vi "Base Json Pretty Formatter.vi"(8 "error in":errorcluster, 10 "ATS Framework Fields in":T1, 11 "json in":string) -> (0 "error out":errorcluster, 3 "json out":string)   [LabVIEW 2022 SP3]
uses:
  Arcadia/Common/Framework/ATS Framework Fields.ctl
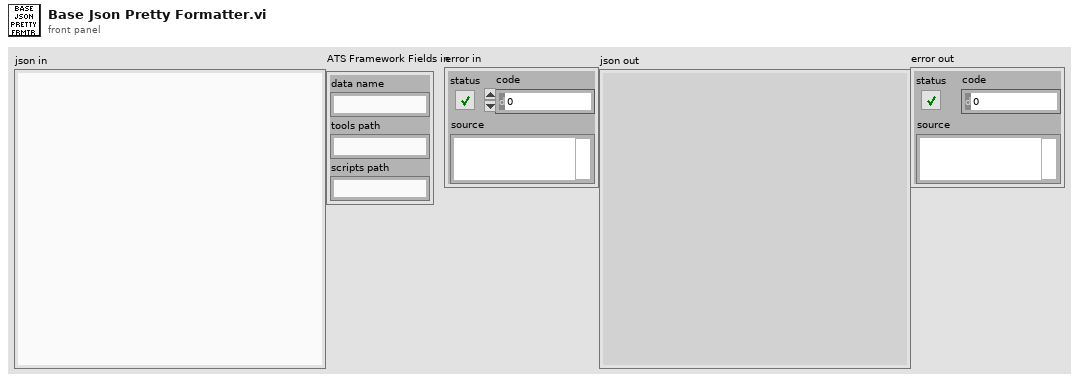
[diagram p1: front panel]
types:
  T1 = typedef "ATS Framework Fields.ctl" = cluster{"data name":string, "tools path":string, "scripts path":string}
  T2 = typedef "Run Tool Output.ctl" = cluster{"cmdline":string, "stdout":string, "stderr":string}
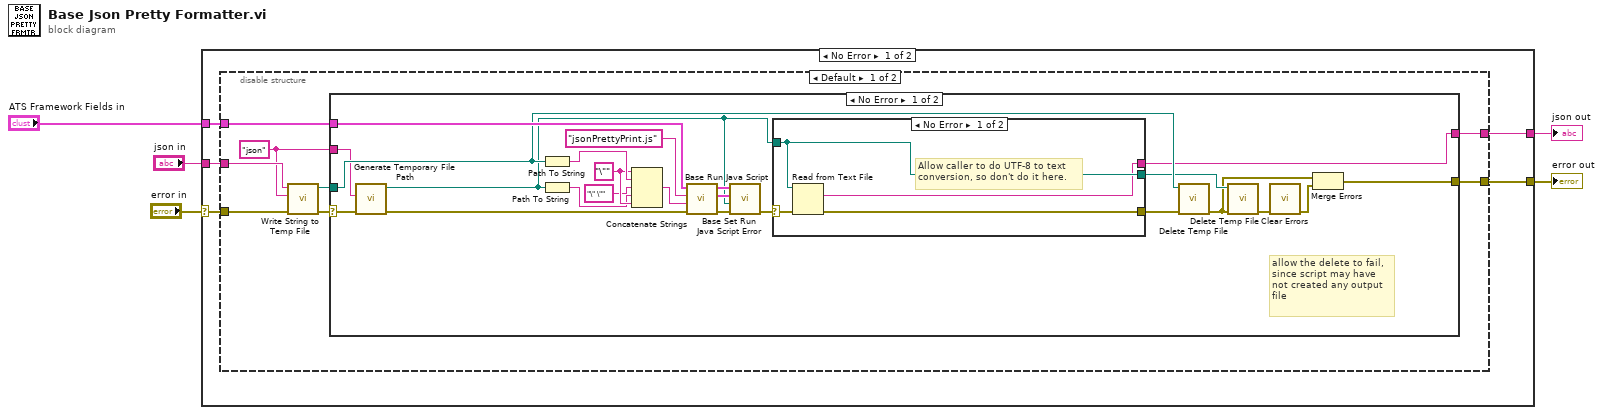
[diagram p0: block diagram]
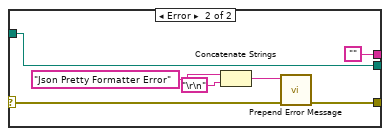
[diagram p2: hidden frame]
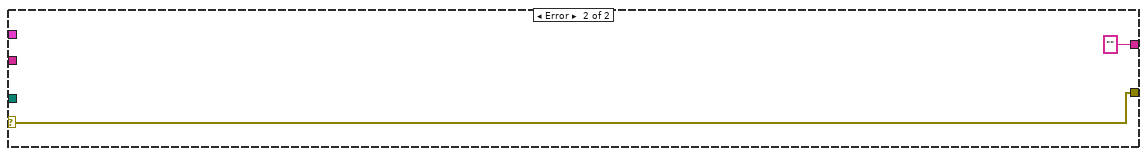
[diagram p3: hidden frame]
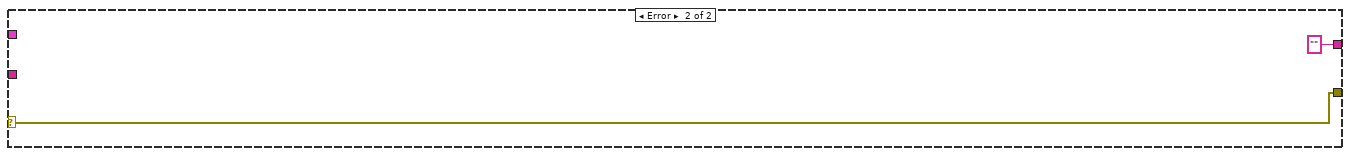
[diagram p5: hidden frame]
diagram:
  n1 = case shown="No Error" "error in" {
    selector: "error in" -> [w7 w58]
    tunnel: [w6 w58] -> w5
    tunnel: "ATS Framework Fields in" -> [w10 _]
    tunnel: [w9 "" ("std out")] -> w2
    tunnel: "json in" -> [w8 _]
    frame No Error {
      n2 = disable-structure shown="Default" {
        disable-tunnel: w10 -> [w18 _]
        disable-tunnel: [w17 w55] -> w9
        disable-tunnel: w8 -> [w16 w55]
        disable-tunnel: w7 -> [w15 w56]
        disable-tunnel: [w14 w56] -> w6
        frame condition #0 (active) {
          w11 = "json" ("file extension in")
          n3 = call "Write String to Temp File.vi"("error in"=w15, "file extension in"=w11, "string in"=w16) -> ("error out"=w12:errorcluster, "file path out"=w13:path)  [unwired: 7 in]
          n4 = case shown="No Error" w12 {
            selector: w12 -> [w31 w54]
            tunnel: w18 -> [w39 _]
            tunnel: [w35 "" ("std out")] -> w17
            tunnel: [w20 w54] -> w14
            tunnel: w13 -> [w36 _]
            tunnel: w11 -> [w29 _]
            frame No Error {
              w27 = "\"" ("string")
              # "allow the delete to fail,\nsince script may have\nnot created any output\nfile"
              n5 = call <vilib>:"Generate Temporary File Path.vi"("error in (no error)"=w31, "Temporary File Extension (tmp)"=w29) -> ("error out"=w30:errorcluster, "Unique Temporary File Path"=w23:path)  [unwired: 8 in]
              n6 = Path To String(path=w36) -> (string=w41:string)
              n7 = Path To String(path=w23) -> (string=w26:string)
              n8 = Concatenate Strings(w27, w41, "\" \"", w26, w27) -> (w40:string)
              n9 = call "Base Run Java Script.vi"("error in"=w30, "script args in"=w40, "script name in"="jsonPrettyPrint.js" ("command line"), "ATS Framework Fields in"=w39) -> ("error out"=w34:errorcluster, "run tool out"=w24:T2, "ATS Framework Fields out"=w32:T1)  [unwired: 1 in]
              n10 = call "Base Set Run Java Script Error.vi"("error in"=w34, "output file in"=w23, "data in"=w24, "ATS Framework Fields in"=w32) -> ("error out"=w33:errorcluster)  [unwired: 3 in]
              n11 = case shown="No Error" w33 {
                selector: w33 -> [w45 w51]
                tunnel: [w43 w50] -> w37
                tunnel: [w42 "" ("std out")] -> w35
                tunnel: w23 -> [w44 w46]
                tunnel: [w44 w46] -> w28
                frame No Error {
                  # "Allow caller to do UTF-8 to text\nconversion, so don't do it here."
                  n12 = Read from Text File(file (use dialog)=w44, error in=w45) -> (text=w42:string, error out=w43:errorcluster)  [unwired: 2 in, 2 out]
                }
                frame Error {
                  n13 = Concatenate Strings("Json Pretty Formatter Error" ("string"), "\r\n") -> (w48:string)
                  n14 = call "Prepend Error Message.vi"("error in"=w51, "message in"=w48) -> ("error out"=w50:errorcluster)  [unwired: 9 in]
                }
              }
              n15 = call "Delete Temp File.vi"("error in"=w37, "file path in"=w36) -> ("error out"=w19:errorcluster)  [unwired: 9 in]
              n16 = call "Delete Temp File.vi"("error in"=w19, "file path in"=w28) -> ("error out"=w21:errorcluster)  [unwired: 9 in]
              n17 = call <vilib>:"Clear Errors.vi"("error in (no error)"=w21) -> ("error out"=w22:errorcluster)  [unwired: 5 in, 1 out]
              n18 = Merge Errors(w19, w22) -> (w20:errorcluster)
            }
            frame Error {
            }
          }
        }
        frame condition #1 {
          # "These oses cannot run jsdb; so for now, just pass the json through unchanged."
        }
      }
    }
    frame Error {
    }
  }
  "error out" <- w5
  "json out" <- w2
